vi "ResultsDB Insert Results Data - Copy.vi"(6 "Results NameList":string, 7 "Total_OK/NG":string, 8 "error in (no error)":errorcluster, 9 "Results List":string, 10 "StationName":string, 11 "MainBarcode":string) -> (0 "error out":errorcluster, 3 "CMD":string)   [LabVIEW 2021, in "SQLite.lvclass"]
doc: "写入每一步的测试结果到Results表格。\n写入原理：先检测已经保存了几个结果数据，然后依次附加到结果数据列上。\n# 2020-6-8 14:05:45"
uses:
  SQLite.lvclass
  Y:/UTP_2023/Source_Public/DataBase/Top DB/Top DB.lvclass
  <vilib>/Utility/error.llb/Trim Whitespace.vi
  SQLite.lvclass/SQLite.ctl
  <userlib>/LabSQL/LabSQL.lvlib
  vi.lib_New/TopPath/TopPath.lvlib
  <userlib>/sushu/sushu.lvlib
panel:
  out "Update CMD 3":string
  out "Update CMD 2":string
  out "Update CMD":string
  out "EmptyResultColumnIndex":i32
  out "FirstRow":string[](array[string])
  out "source":string
  out "match substring":string
  out "number (0 to 1)":dbl
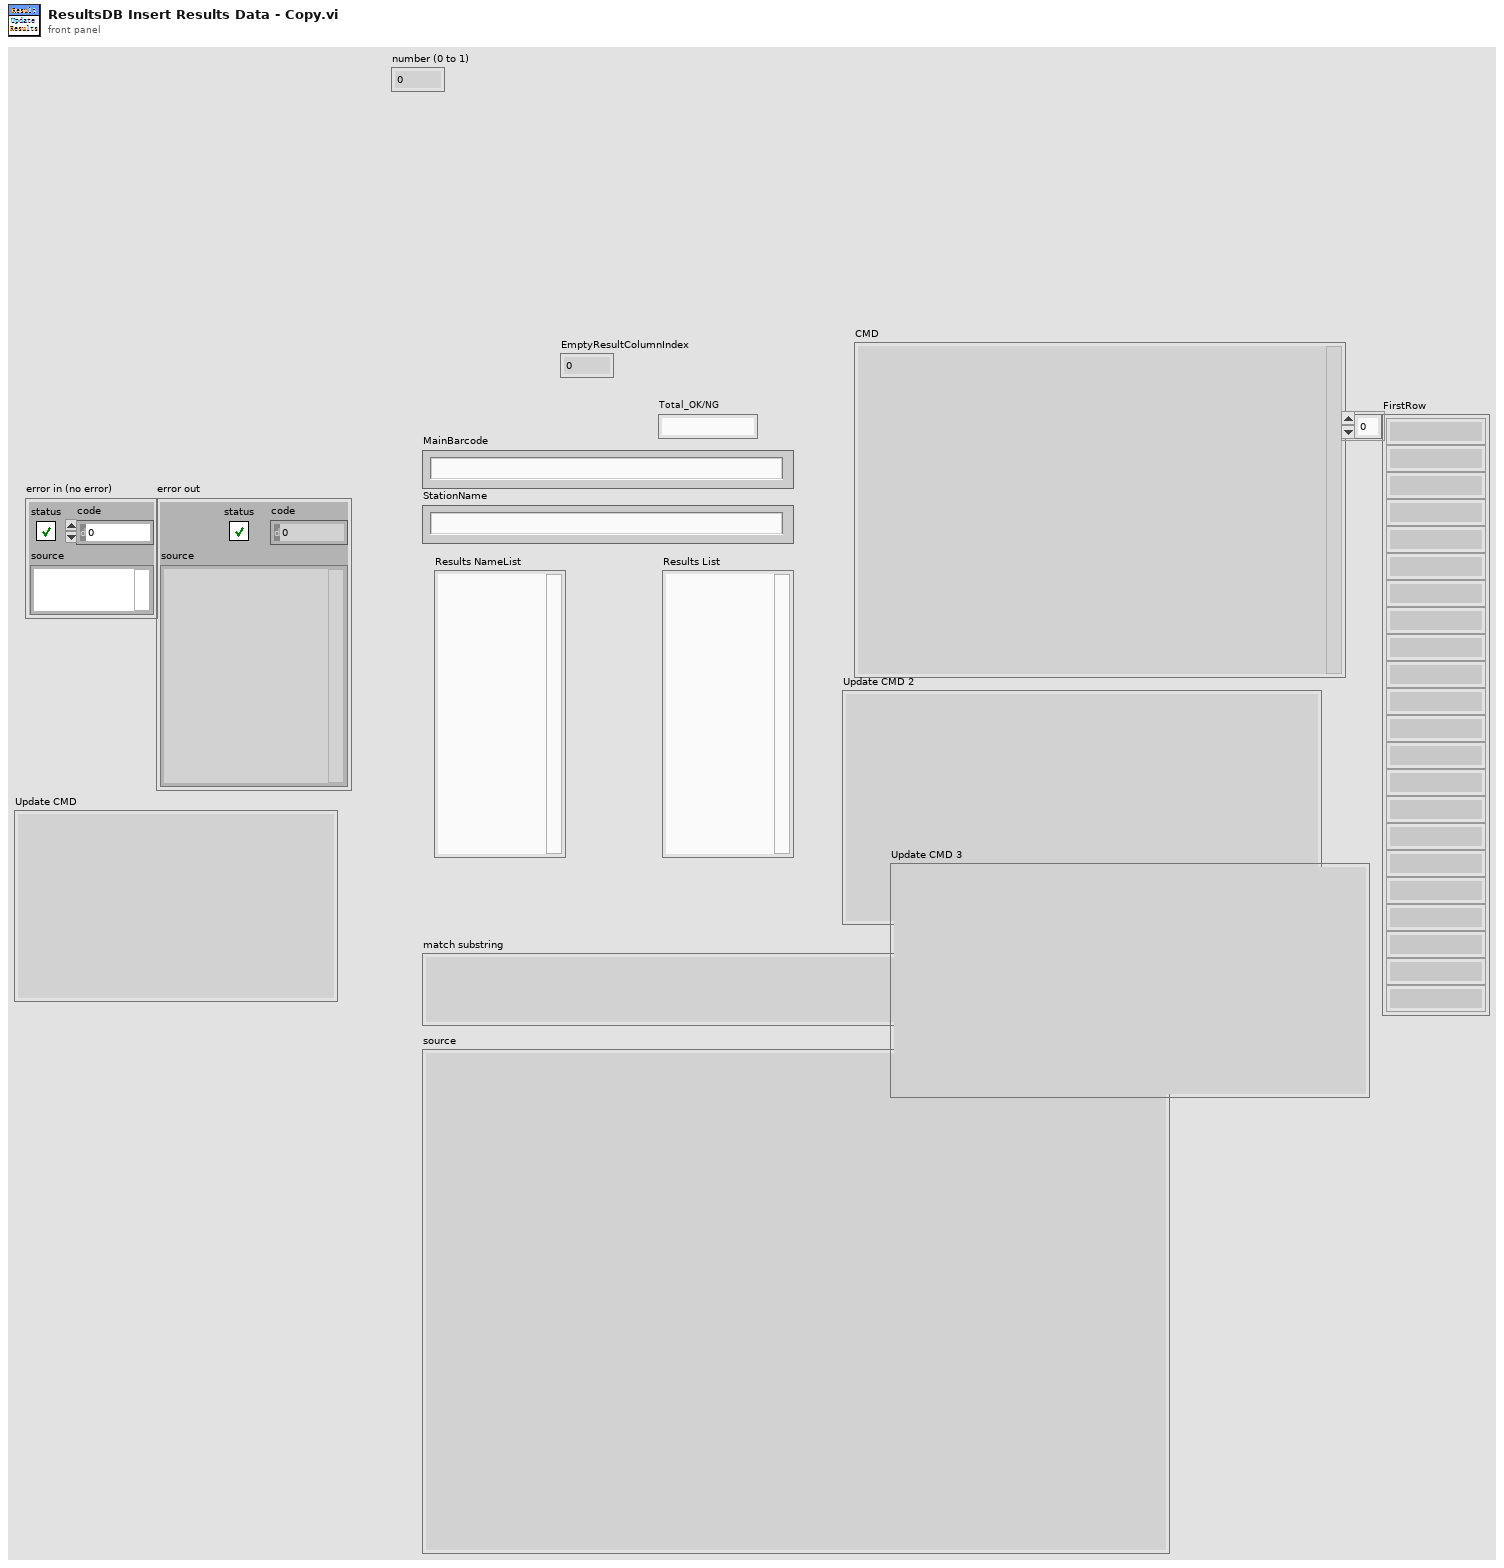
[diagram p1: front panel]
types:
  T1 = cluster{"Core":cluster{"Current VI Reference":refnum<vi>, "Close Panel on Exit?":bool}, "VI Name":string, "Row Numbers":string, "Update?":bool, "CMD":string, "ResultStartindex":i32, "EmptyResultColumnIndex":i32}
  T2 = enum16{"Other", "SQL2008", "SQLite", "Access", "MySQL"}
  T3 = typedef "TopPath.lvlib/Top Path.ctl" = cluster{"LV Source":path, "FilePath":path, "Data":path}
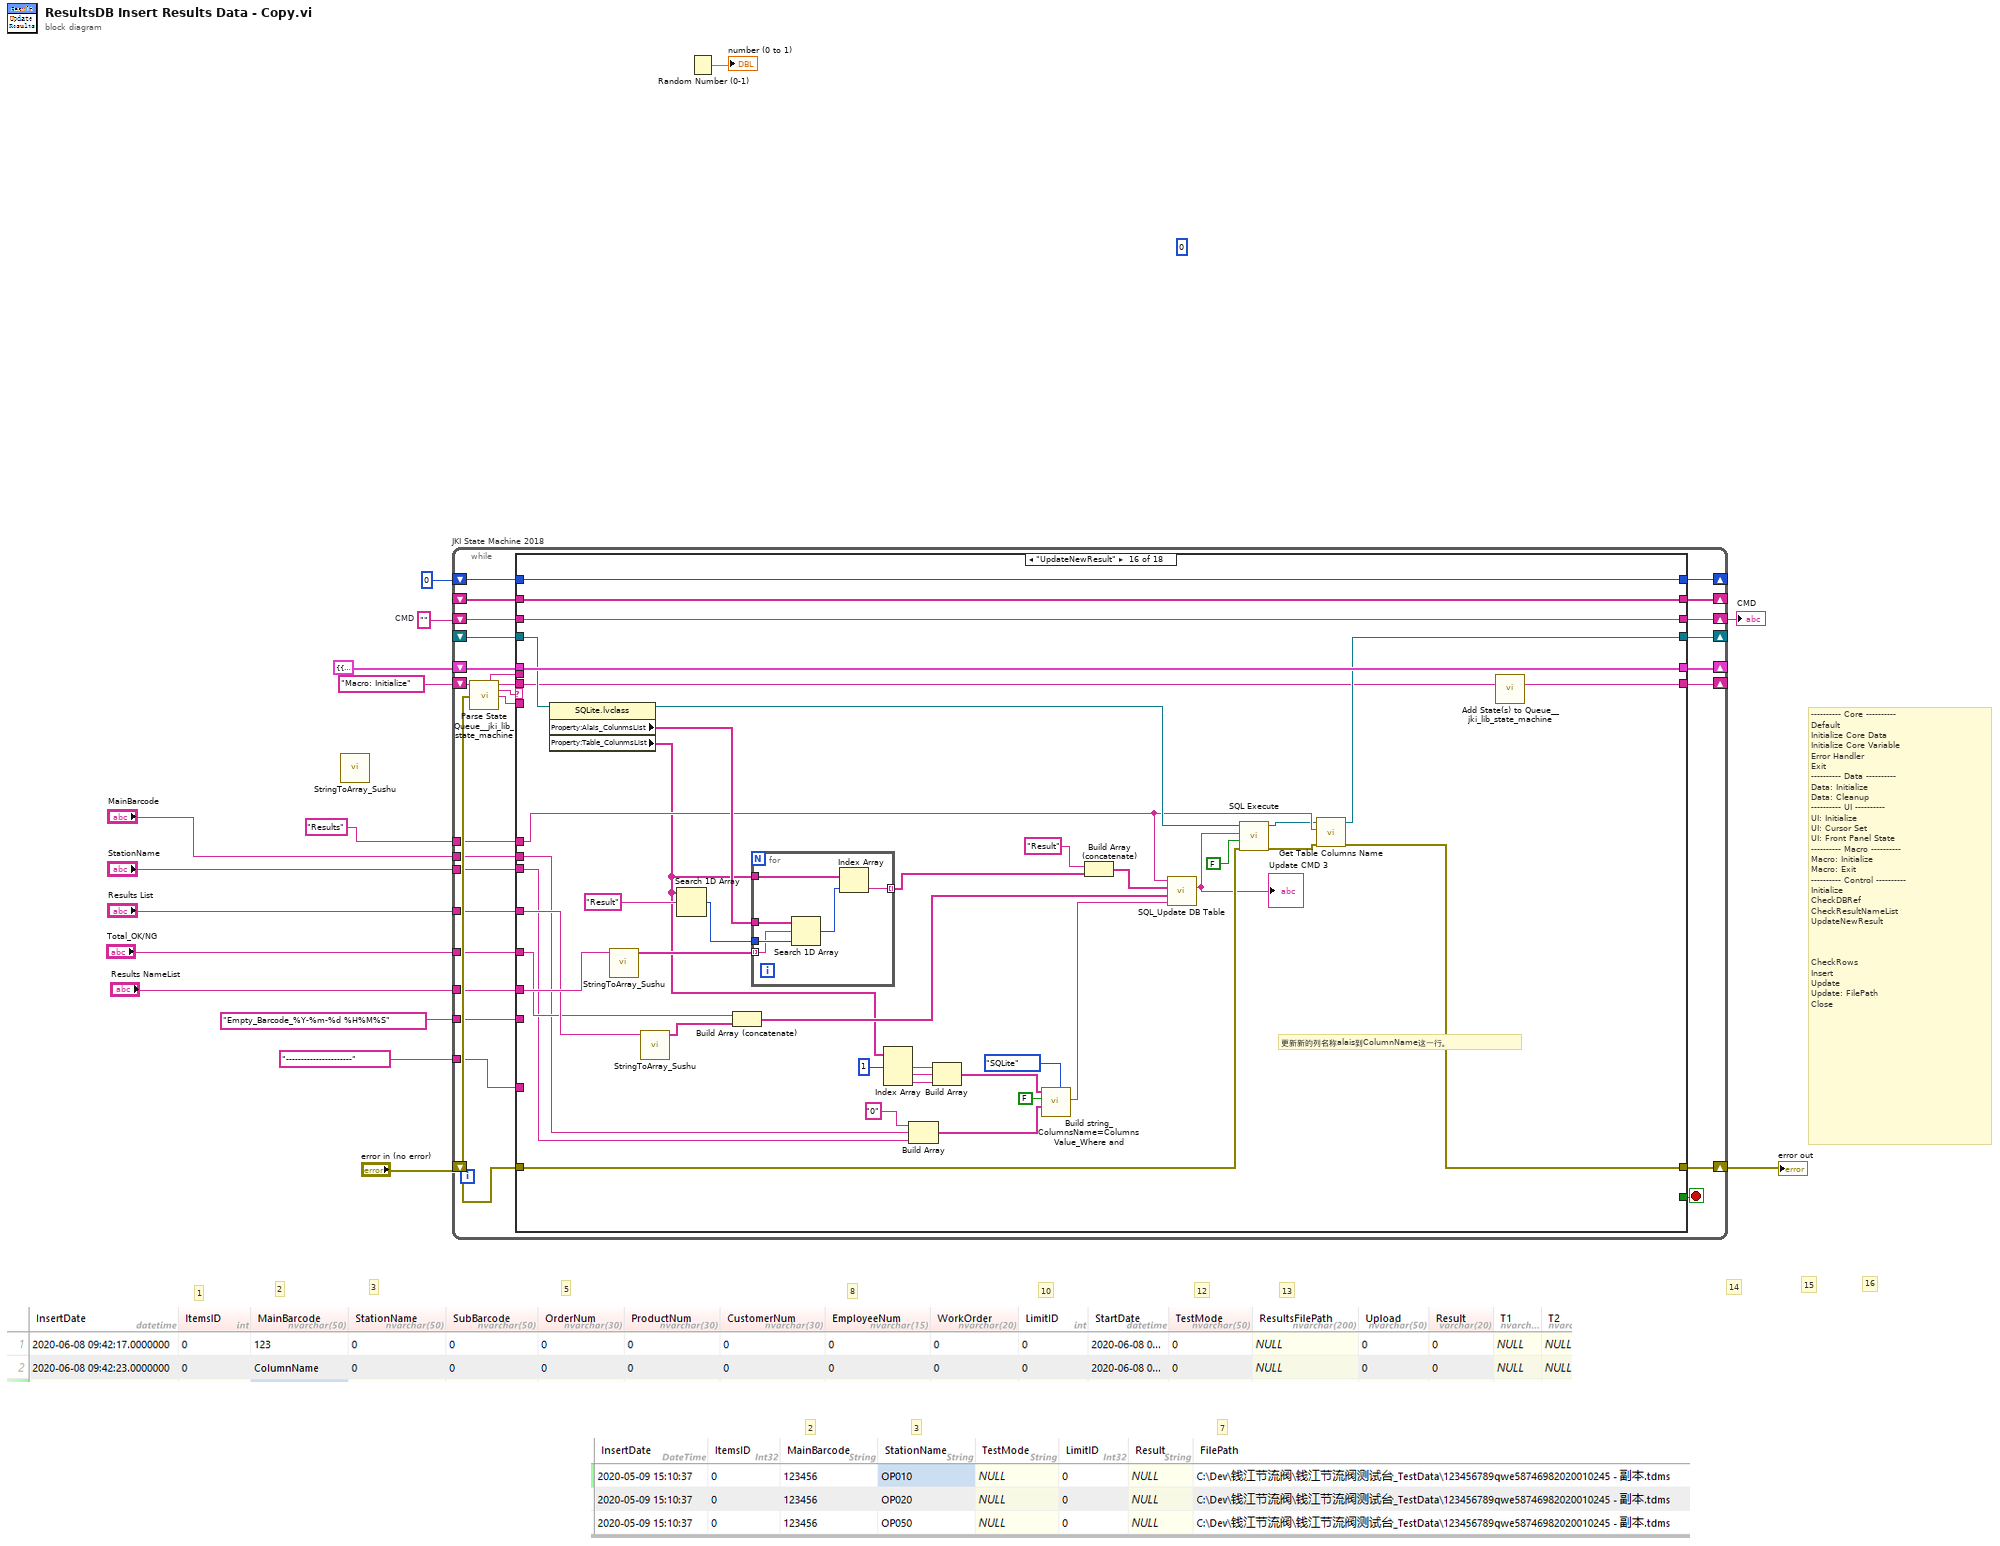
[diagram p0: block diagram]
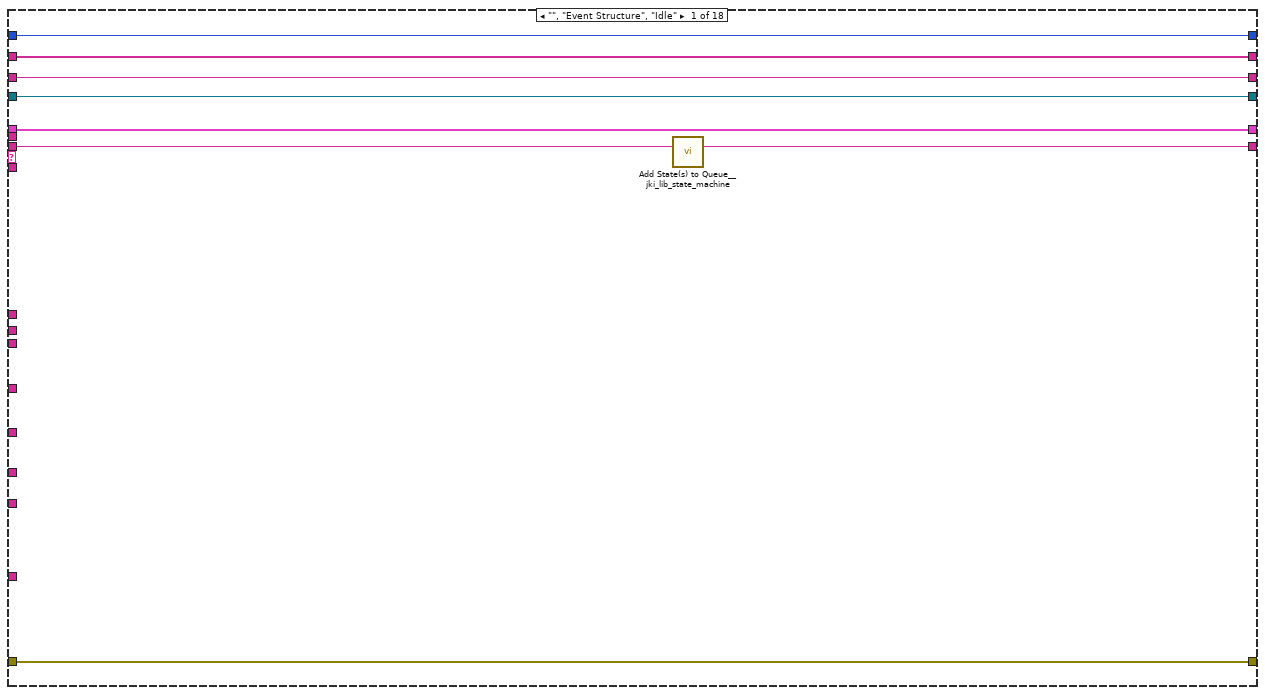
[diagram p2: hidden frame]
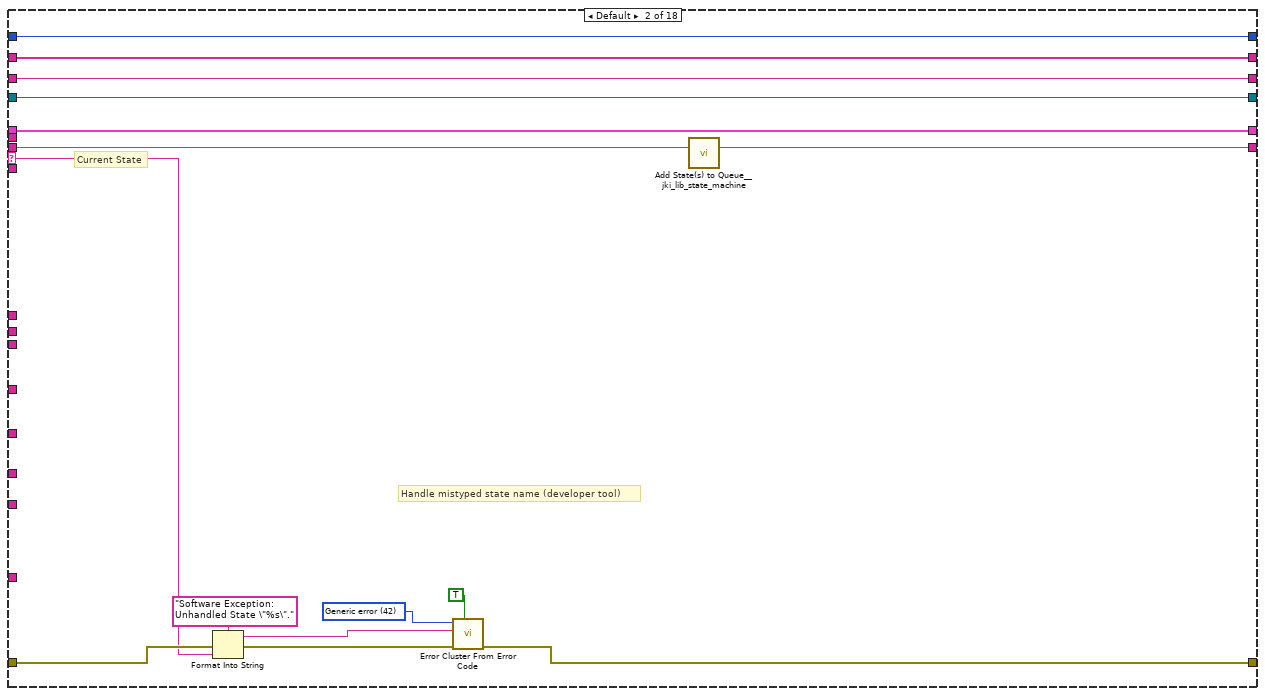
[diagram p3: hidden frame]
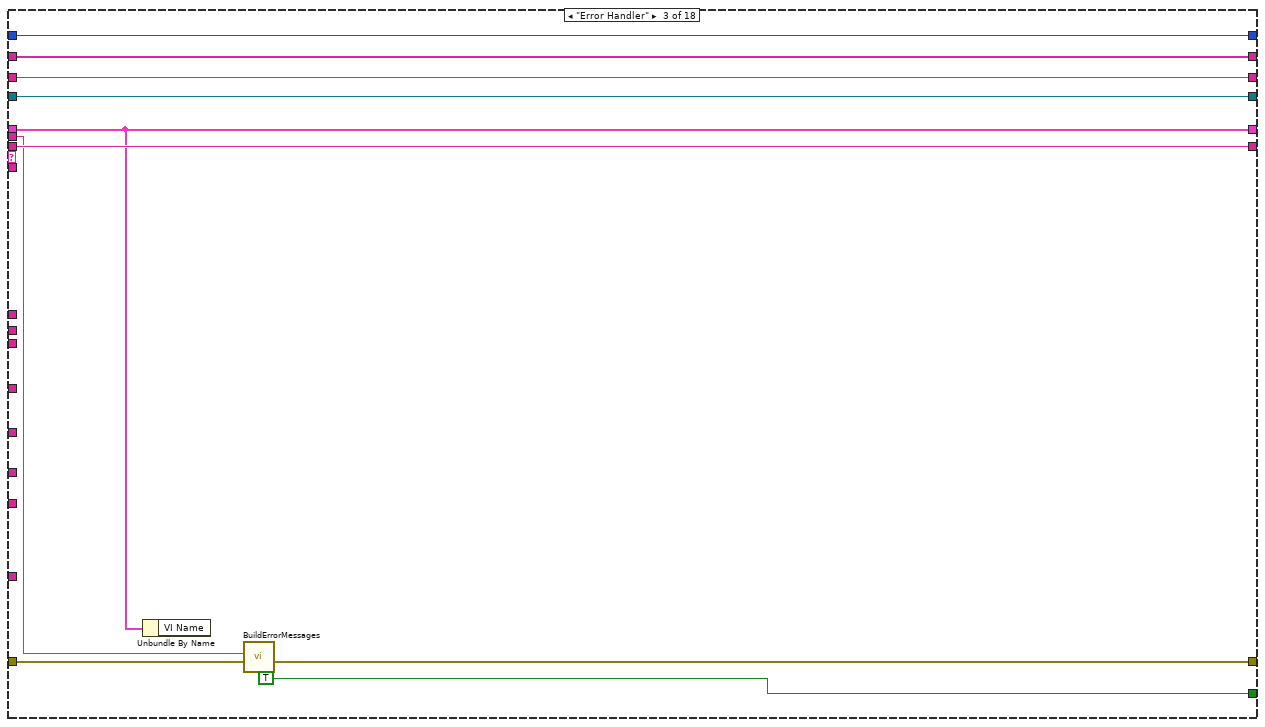
[diagram p4: hidden frame]
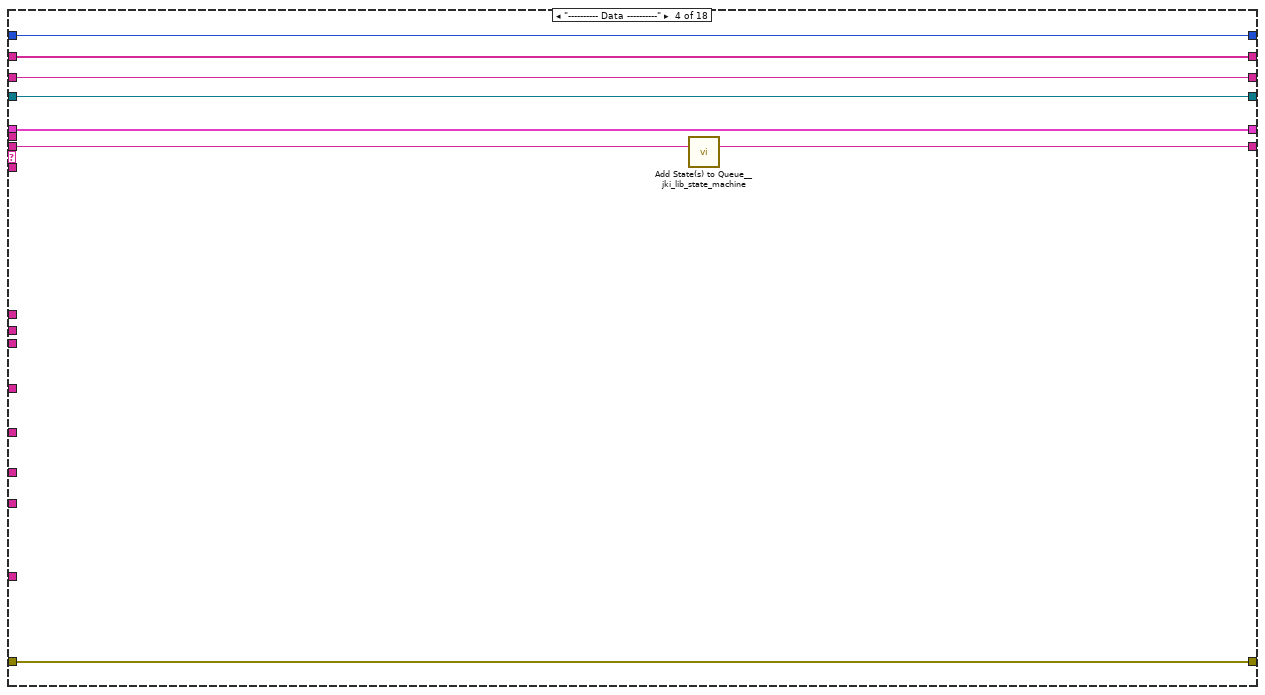
[diagram p5: hidden frame]
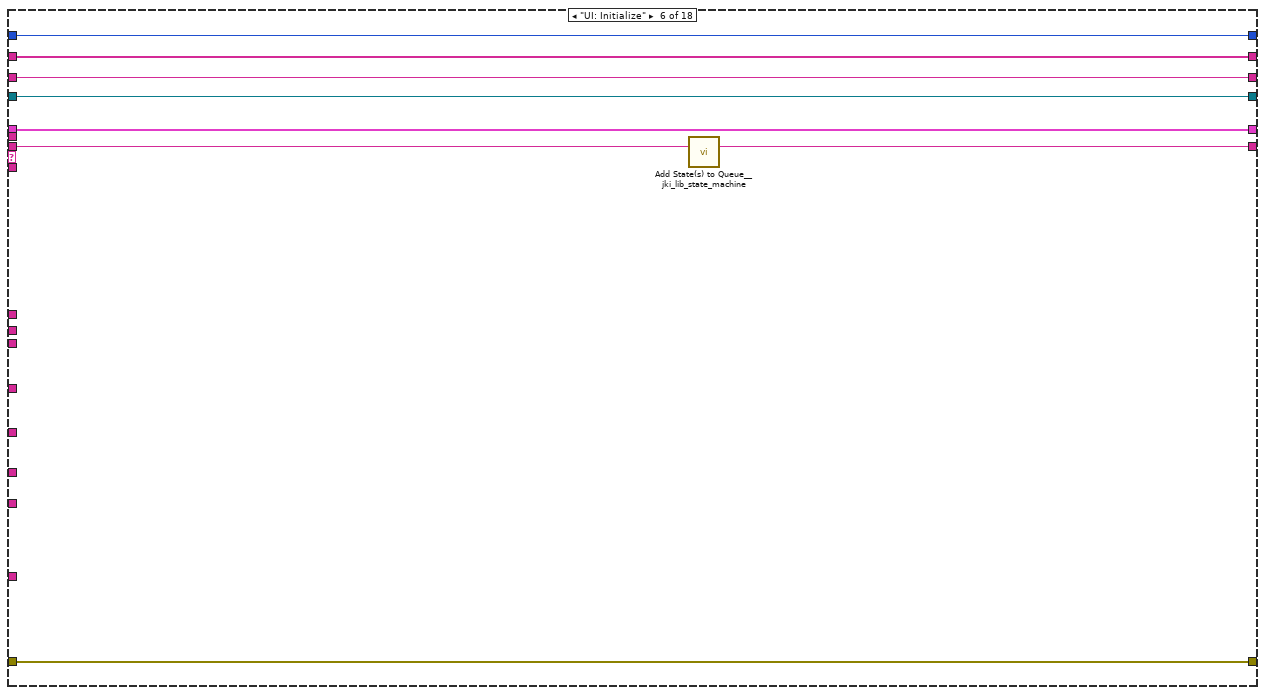
[diagram p7: hidden frame]
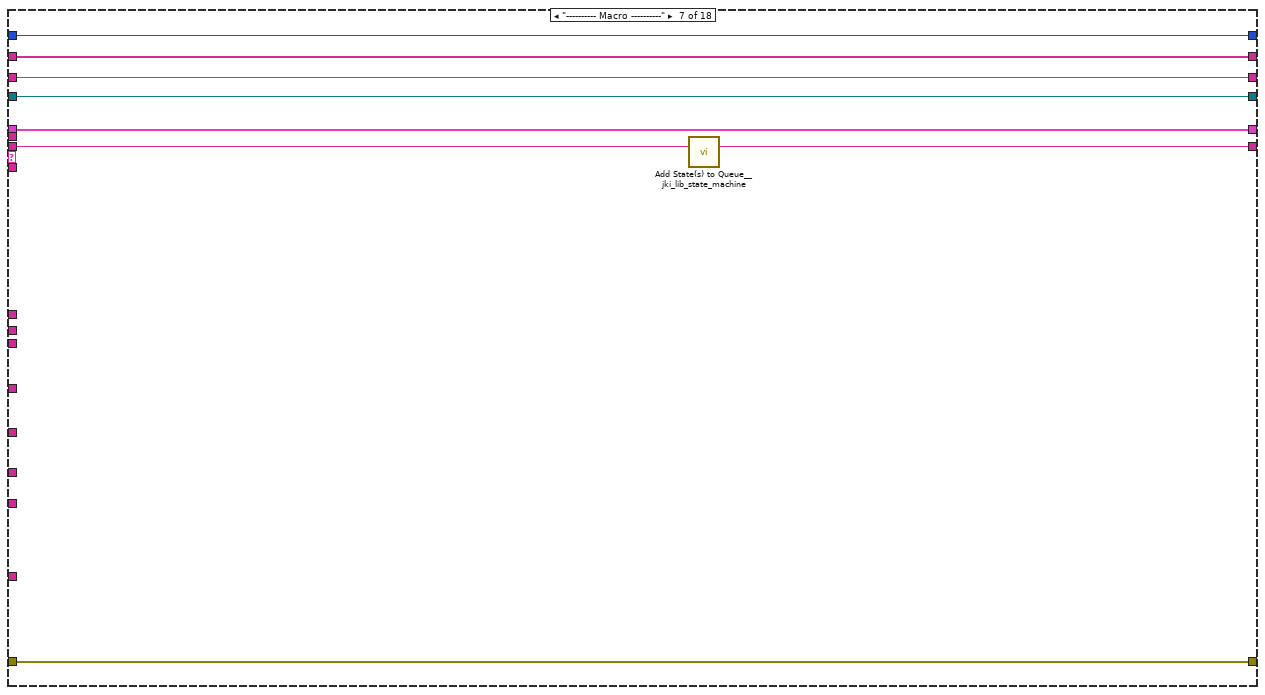
[diagram p8: hidden frame]
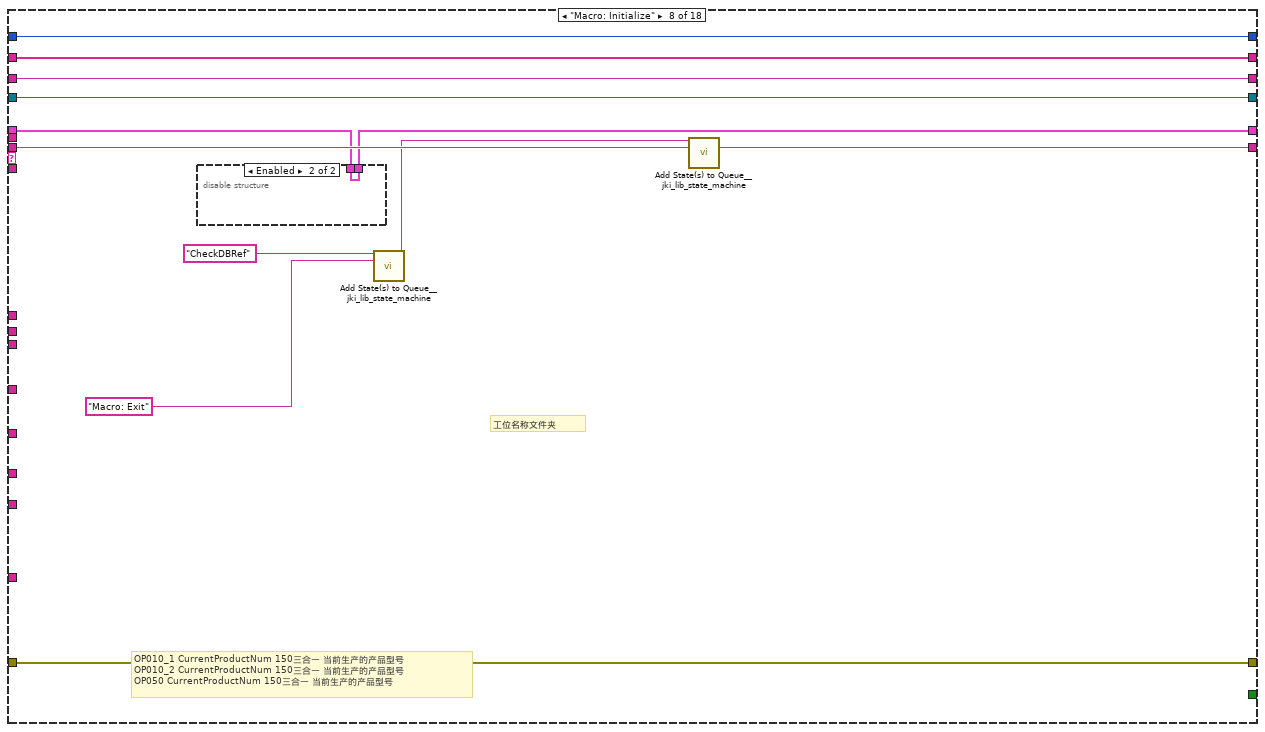
[diagram p9: hidden frame]
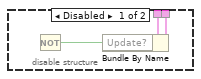
[diagram p10: hidden frame]
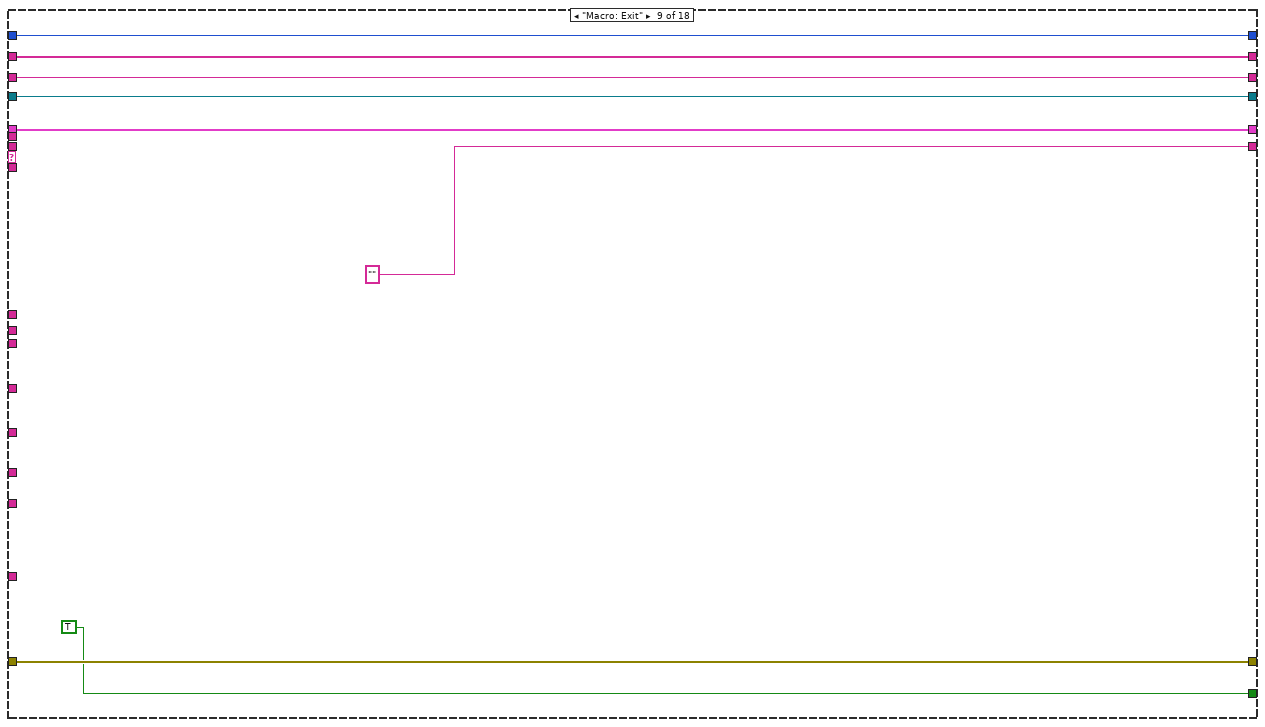
[diagram p11: hidden frame]
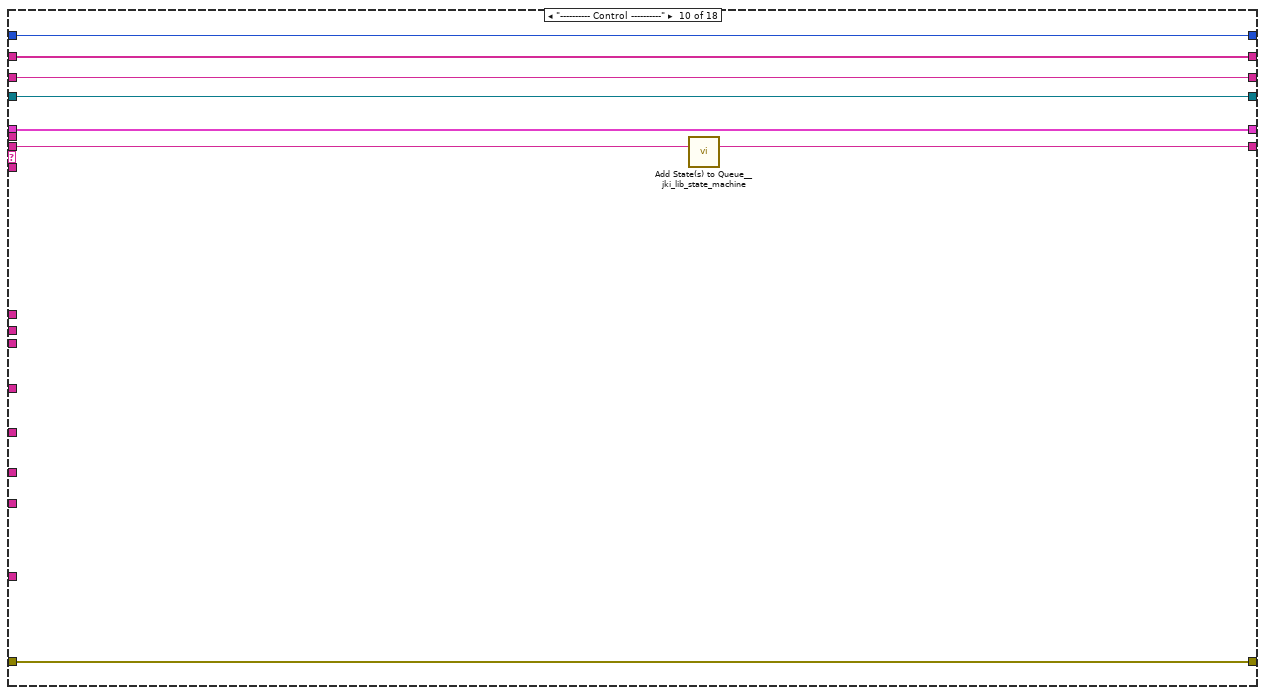
[diagram p12: hidden frame]
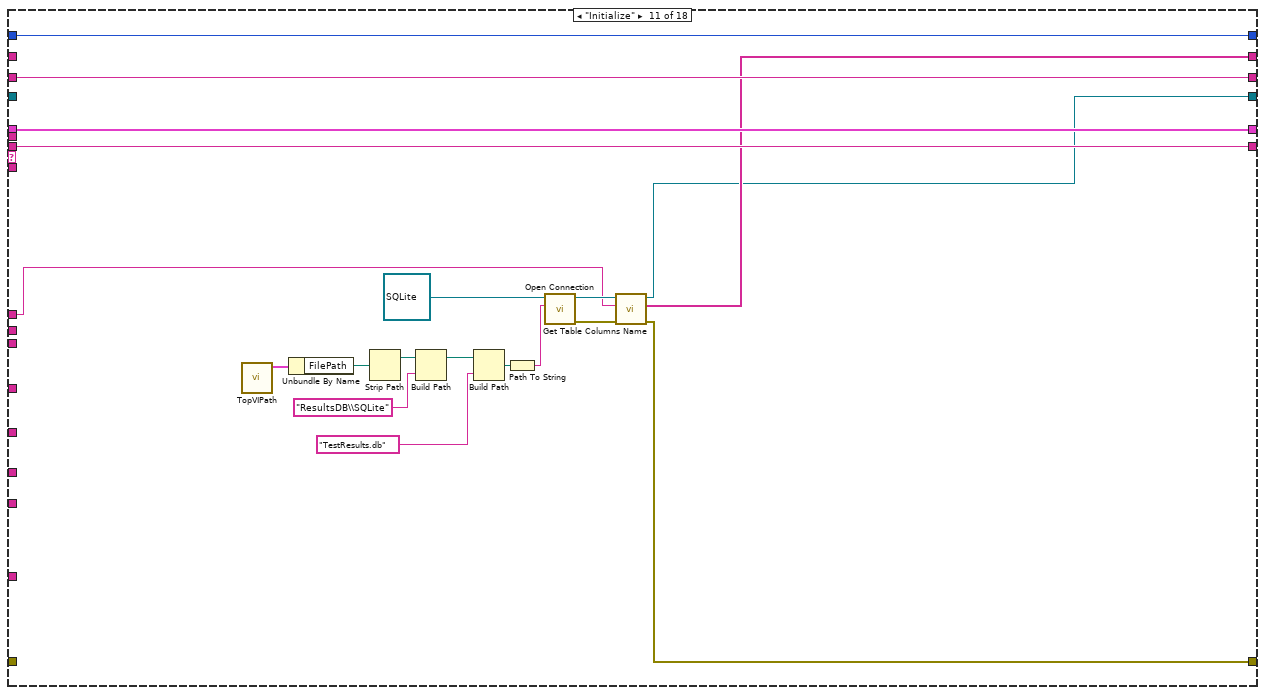
[diagram p13: hidden frame]
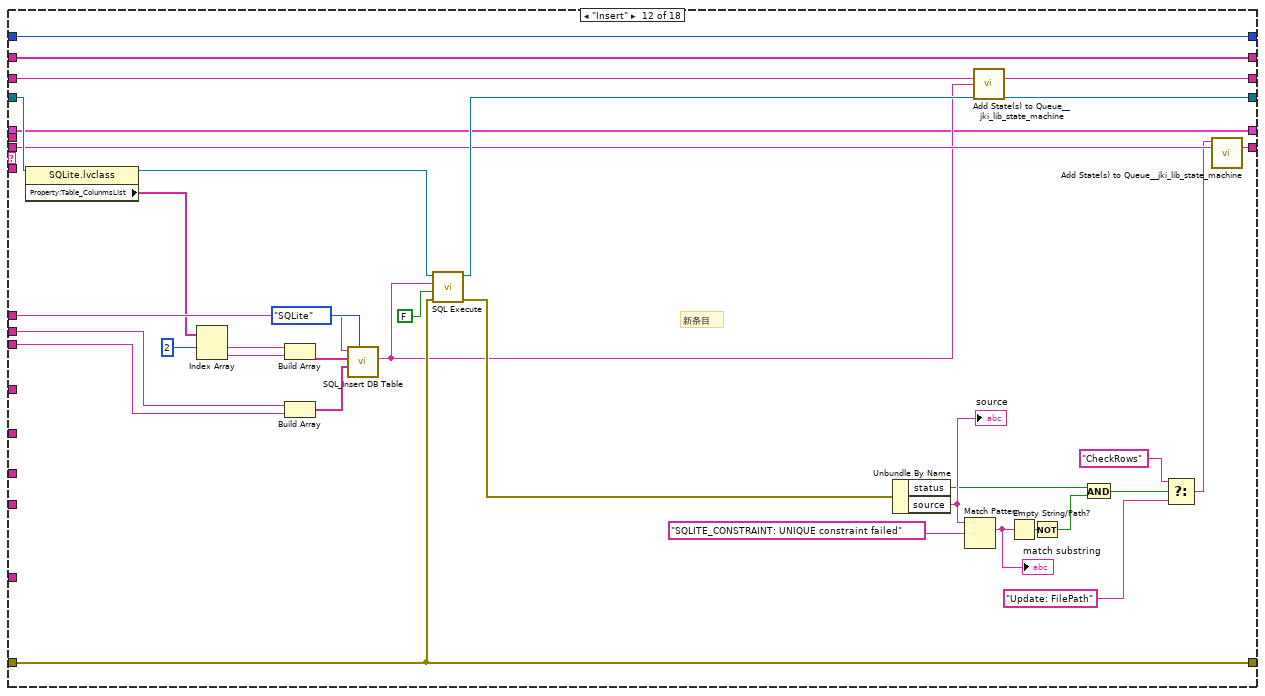
[diagram p14: hidden frame]
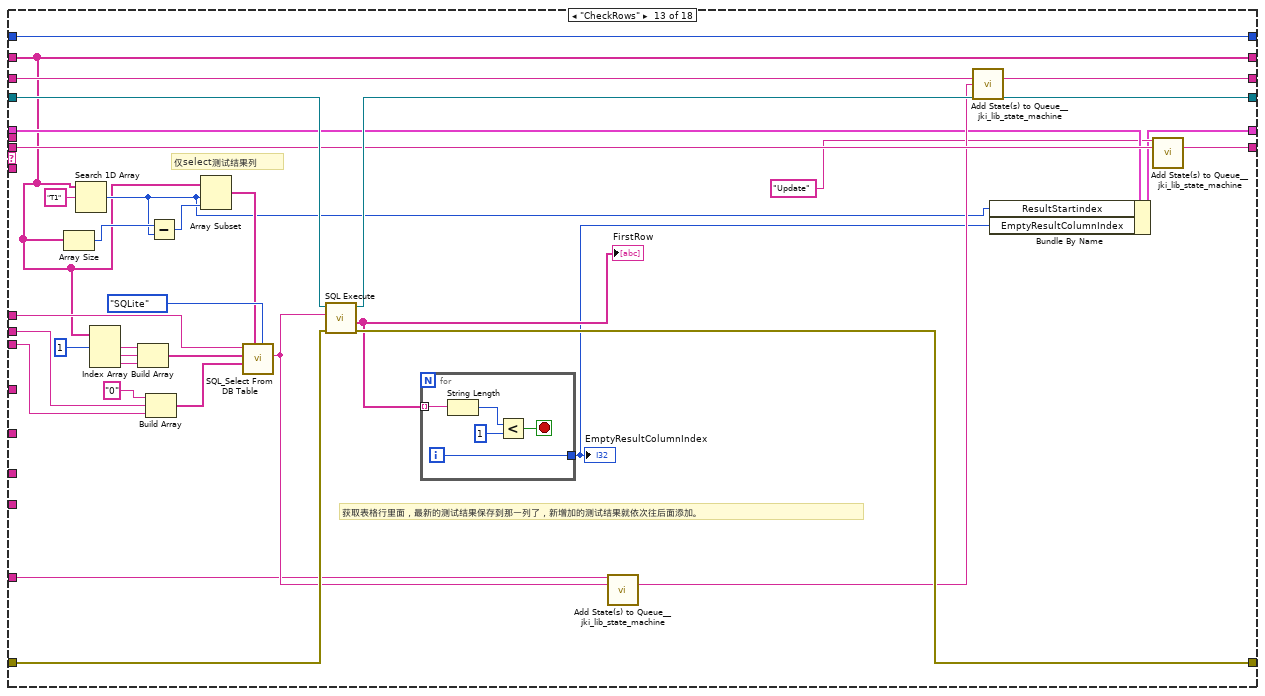
[diagram p15: hidden frame]
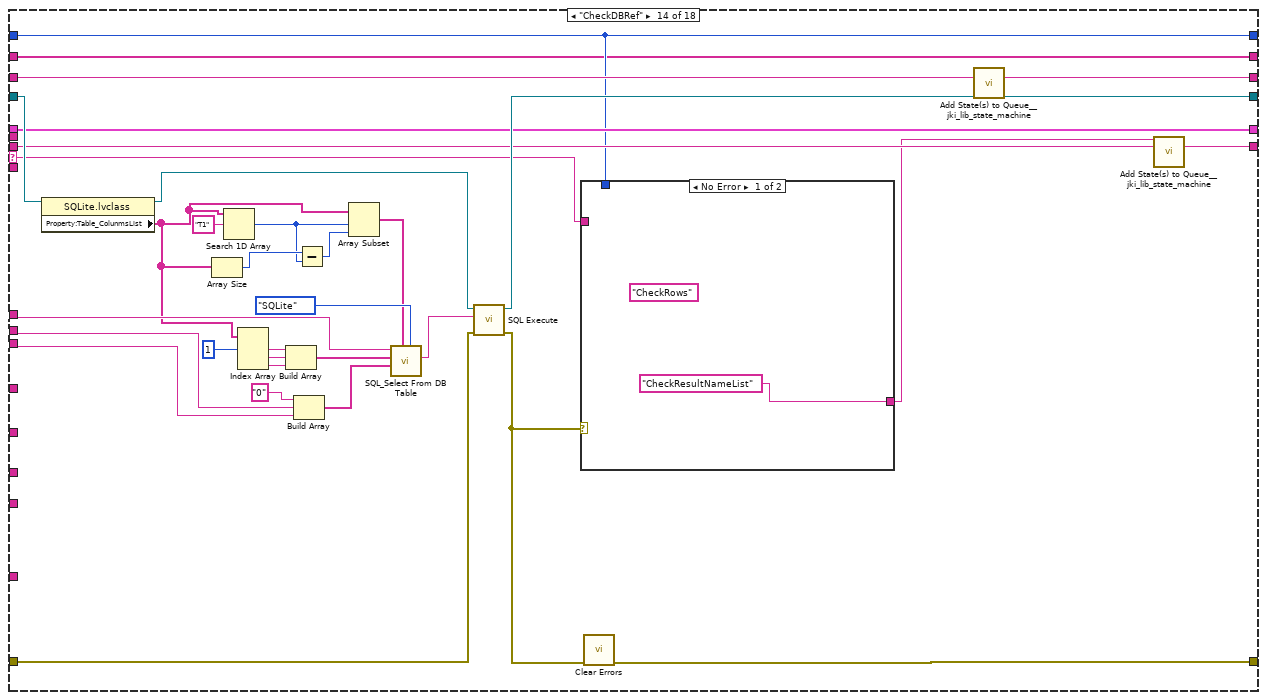
[diagram p16: hidden frame]
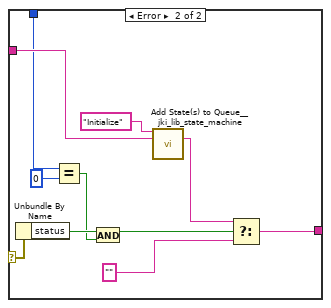
[diagram p17: hidden frame]
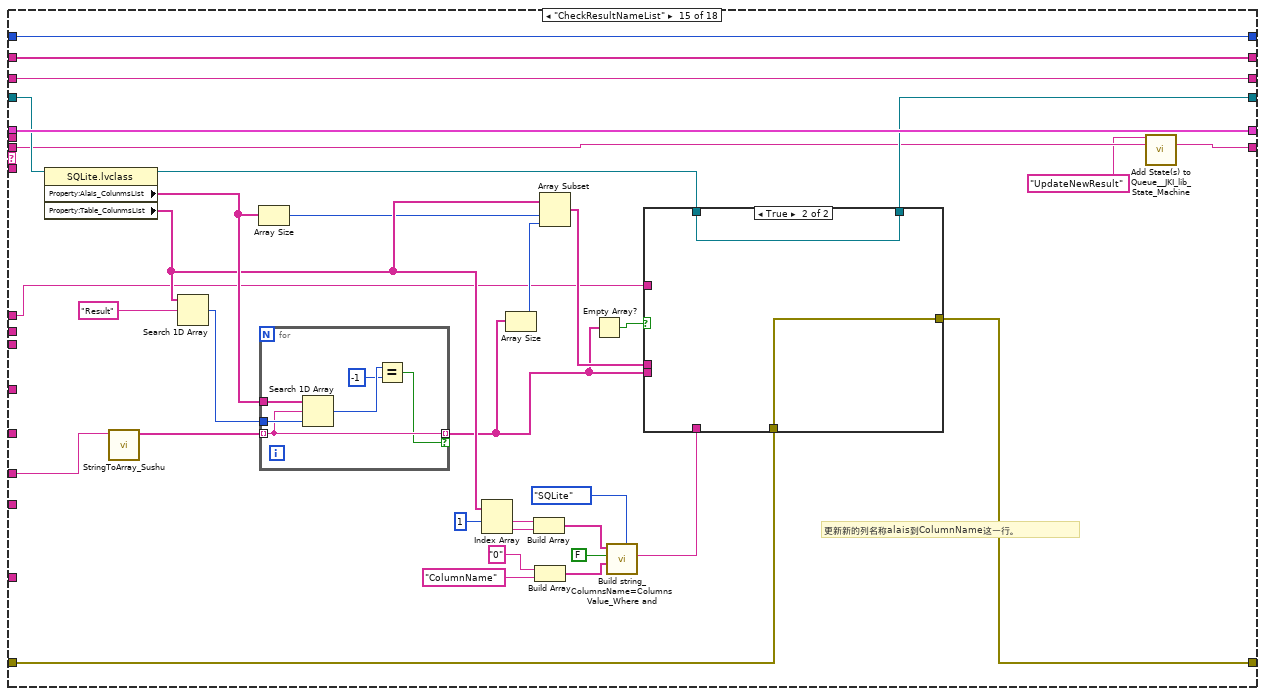
[diagram p18: hidden frame]
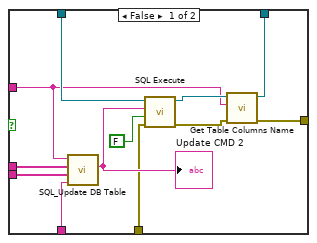
[diagram p19: hidden frame]
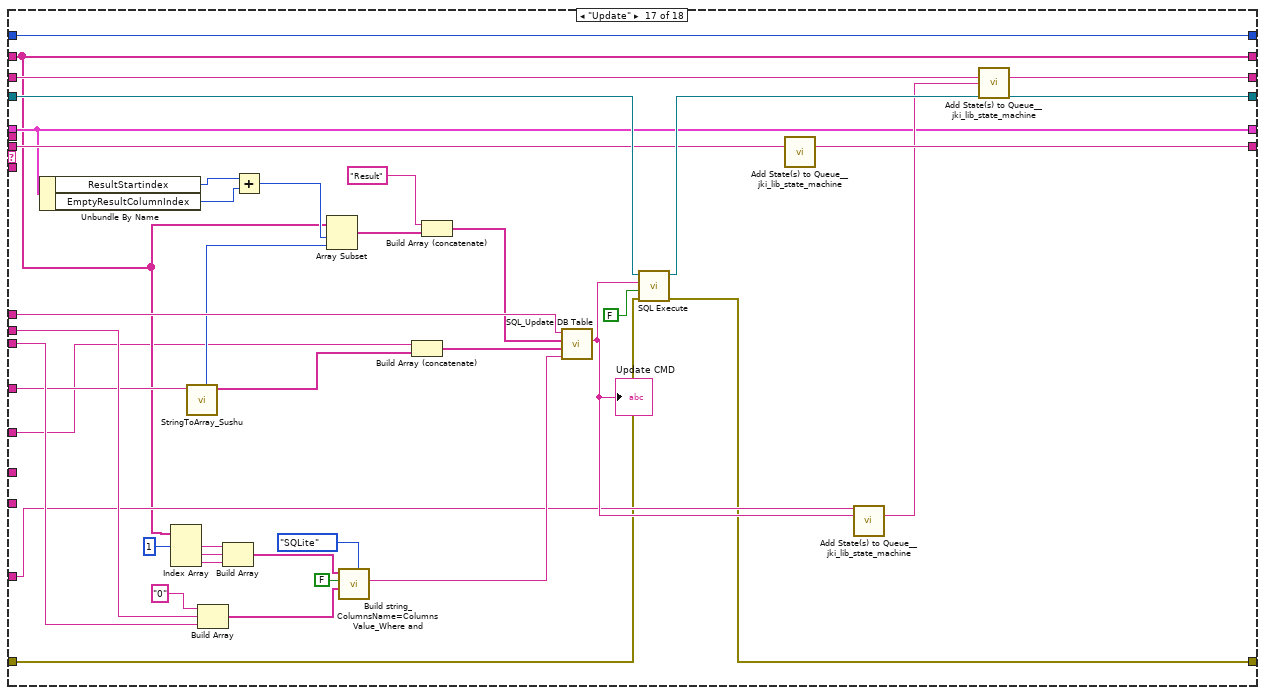
[diagram p20: hidden frame]
diagram:
  w9 = ""  # CMD
  (unwired) 0 ("index (row)")
  # "16"
  # "15"
  # "14"
  # "13"
  # "12"
  # "10"
  # "8"
  # "5"
  # "3"
  # "2"
  # "1"
  # "---------- Core ----------\nDefault\nInitialize Core Data\nInitialize Core Variable\nError Handler\nExit\n---------- Data ----------\nData: Initialize\nData: Cleanup\n---------- UI ----------\nUI: Initialize\nUI: Cursor Set\nUI: Front Panel State\n---------- Macro ----------\nMacro: Initialize\nMacro: Exit\n---------- Control ----------\nInitialize\nCheckDBRef\nCheckResultNameList\nUpdateNewResult\n\n\n\nCheckRows\nInsert\nUpdate\nUpdate: FilePath\nClose"
  # "7"
  # "3"
  # "2"
  n1 = call <userlib>:"StringToArray_Sushu.vi"() -> ()  [unwired: 8 in, 4 out]
  n2 = while "JKI State Machine 2018" {
    shift-right: [w37] -> _
    shift-left: T1 {"Core"={"Current VI Reference"=refnum, "Close Panel on Exit?"=FALSE}, "VI Name"="", "Row Numbers"="", "Update?"=FALSE, "CMD"="", "ResultStartindex"=0, "EmptyResultColumnIndex"=0} ("Data") -> [w36]
    shift-right: [w40] -> w3
    shift-left: "error in (no error)" -> [w35]
    shift-right: [w39] -> _
    shift-left: "Macro: Initialize" -> [w41]
    shift-right: [w33] -> _
    shift-left: _ -> [w34]
    tunnel: "StationName" -> [w31]
    tunnel: "MainBarcode" -> [w30]
    tunnel: "Results" ("TableName") -> [w29]
    tunnel: "Empty_Barcode_%Y-%m-%d %H%M%S" ("time format string (%c)") -> [w28]
    shift-right: [w27] -> w7
    shift-left: w9 -> [w26]
    tunnel: "----------------------" ("State(s) in (\"\")") -> [w25]
    tunnel: "Results List" -> [w24]
    shift-right: [w22] -> _
    shift-left: _ -> [w23]
    shift-right: [w21] -> _
    shift-left: 0 ("y") -> [w20]
    tunnel: "Total_OK/NG" -> [w19]
    tunnel: "Results NameList" -> [w17]
    stop <- w38 stop-if-true
    n3 = call <vilib>:"Parse State Queue__jki_lib_state_machine.vi"("State Queue"=w41, "Error In (no error)"=w35) -> ("Previous State"=w18:string, "Remaining States"=w43:string, "Current State"=w32:string, "Arguments"=w42:string)  [unwired: 10 in]
    n4 = case shown="\"UpdateNewResult\"" w32 {
      selector: w32 -> [_ w56 _ _ _ _ _ _ _ _ _ _ _ w239 _ _ _ _]
      tunnel: w43 -> [w51 w60 w75 w84 w88 w99 w107 w119 _ w139 w158 w170 w214 w252 w278 w355 w409 w425]
      tunnel: w42 -> [_ _ _ _ _ _ _ _ _ _ _ _ _ _ _ _ _ _]
      tunnel: w36 -> [w48 w58 w73 w81 w89 w97 w104 w115 w130 w136 w157 w163 w200 w241 w310 w371 w392 w424]
      tunnel: [w49 w62 w70 w82 w91 w96 w105 w116 w131 w137 w143 w180 w212 w235 w283 w358 w384 w419] -> w40
      tunnel: w35 -> [w49 w61 w71 w82 w91 w96 w105 w116 w131 w137 _ w180 w213 w251 w301 w362 w385 w420]
      tunnel: [w50 w59 w75 w83 w88 w98 w106 w118 "" w138 w158 w171 w215 w253 w279 w356 w410 w425] -> w39
      tunnel: [_ _ TRUE _ _ _ _ _ TRUE _ _ _ _ _ _ _ _ _] -> w38
      tunnel: [w48 w58 w73 w81 w89 w97 w104 w111 w130 w136 w157 w163 w197 w241 w310 w371 w392 w424] -> w37
      tunnel: w34 -> [w47 w55 w74 w80 w90 w95 w103 w117 w129 w135 _ w183 w217 w255 w309 w370 w413 w418]
      tunnel: [w47 w55 w74 w80 w90 w95 w103 w117 w129 w135 w140 w182 w216 w254 w284 w359 w412 w417] -> w33
      tunnel: w18 -> [_ _ w72 _ _ _ _ _ _ _ _ _ _ _ _ _ _ _]
      tunnel: w31 -> [_ _ _ _ _ _ _ _ _ _ _ w184 w218 w256 _ w331 w414 _]
      tunnel: w30 -> [_ _ _ _ _ _ _ _ _ _ _ w185 w219 w257 _ w332 w415 _]
      tunnel: w29 -> [_ _ _ _ _ _ _ _ _ _ w144 w186 w220 w258 w282 w357 w416 _]
      tunnel: w28 -> [_ _ _ _ _ _ _ _ _ _ _ _ _ _ _ _ _ _]
      tunnel: w26 -> [w46 w54 w69 w79 w87 w94 w102 w112 w126 w134 w156 w166 w210 w249 w308 w369 w397 w423]
      tunnel: [w46 w54 w69 w79 w87 w94 w102 w112 w126 w134 w156 w165 w211 w250 w308 w369 w398 w423] -> w27
      tunnel: w25 -> [_ _ _ _ _ _ _ _ _ _ _ _ w207 _ _ _ w394 _]
      tunnel: w24 -> [_ _ _ _ _ _ _ _ _ _ _ _ _ _ _ w350 w393 _]
      tunnel: w23 -> [w45 w53 w68 w78 w86 w93 w101 w109 w125 w133 _ w160 w194 w233 w307 w368 w383 w422]
      tunnel: [w45 w53 w68 w78 w86 w93 w101 w109 w125 w133 w141 w160 w194 w233 w307 w368 w383 w422] -> w22
      tunnel: w20 -> [w44 w52 w67 w77 w85 w92 w100 w108 w124 w132 w142 w162 w193 w238 w306 w367 w382 w421]
      tunnel: [w44 w52 w67 w77 w85 w92 w100 w108 w124 w132 w142 w162 w193 w238 w306 w367 w382 w421] -> w21
      tunnel: w19 -> [_ _ _ _ _ _ _ _ _ _ _ _ _ _ _ w348 w380 _]
      tunnel: w17 -> [_ _ _ _ _ _ _ _ _ _ _ _ _ _ w285 w360 _ _]
      frame "", "Event Structure", "Idle" {
        n5 = call <vilib>:"Add State(s) to Queue__jki_lib_state_machine.vi"("State(s) in (\"\")"=w51) -> ("States Out"=w50:string)  [unwired: 14 in]
      }
      frame Default {
        w65 = 42 items=["No error", "Argument error", "Memory is full", "Out of zone", "End of file", "File already open", "Generic file I/O error", "File not found", "File permission error", "Disk is full", "Duplicate path", "Too many files open", "System feature not enabled", "Resource file not found", "Cannot add resource", "Resource not found", "Image not found", "Image memory error", "Pen does not exist", "Config type invalid", "Config token not found", "Config parse error", "Config memory error", "Bad external code format", "Bad external code offset", "External code not present", "Null window", "Destroy window error", "Null menu", "Print aborted", "Bad print record", "Print driver error", "Windows error during printing", "Memory error during printing", "Print dialog error", "Generic print error", "Invalid device refnum", "Device not found", "Device parameter error", "Device unit error", "Cannot open device", "Device call aborted", "Generic error", "Cancelled by user", "Object ID too low", "Object ID too high", "Object not in heap", "Unknown heap", "Unknown object (invalid DefProc)", "Unknown object (DefProc not in table)", "Message out of range", "Invalid (null) method", "Unknown message", "Manager call not supported", "Bad address", "Network operation in progress", "Network operation timed out", "Connection is busy", "Network attribute not supported", "Network error", "Address in use", "System out of memory", "Connection aborted", "Connection refused", "Not connected", "Already connected", "Connection closed", "Initialization error (interapplication manager)", "Bad occurrence", "Wait on unbound occurrence handler", "Occurrence queue overflow", "Datalog type conflict", "Unused", "Unrecognized type (interapplication manager)", "Memory corrupt", "Failed to make temporary DLL", "Old CIN version", "Drag socket not found", "Failed to load drop-object", "Failed to register OLE object", "Failed to release OLE object", "Format specifier type mismatch", "Unknown format specifier", "Too few format specifiers", "Too many format specifiers", "Scan failed", "Newer CIN version", "Error converting to variant", "Runtime menu error", "Password tampered", "Variant attribute not found", "Incompatible variant data type", "Event data is not available", "Event Store is not present", "Occurrence is not found", "Event Queue is not created", "Event info is not available", "Refnum passed is NULL", "Error retrieving Class GUID", "Error retrieving CoClass GUID", "Error retrieving TypeLib GUID.", "Bad built application magic bytes.", "Specific driver is different from the specific driver associated with the Logical Name.", "There is no session opened to the class driver.", "Max Error", "MAX - Error with config objects", "MAX - Error loading configuration", "MAX - Group not supported"]
        # "Current State"
        # "Handle mistyped state name (developer tool)"
        n6 = Format Into String(format string="Software Exception: Unhandled State \"%s\"." ("message"), error in=w61, w56) -> (resulting string=w64:string, error out=w63:errorcluster)  [unwired: 1 in]
        n7 = call <vilib>:"Error Cluster From Error Code.vi"("show call chain? (False)"=TRUE, "error in (no error)"=w63, "error message (\"\")"=w64, "error code (0)"=w65) -> ("error out"=w62:errorcluster)  [unwired: 5 in]
        n8 = call <vilib>:"Add State(s) to Queue__jki_lib_state_machine.vi"("State(s) in (\"\")"=w60) -> ("States Out"=w59:string)  [unwired: 14 in]
      }
      frame "Error Handler" {
        n9 = Unbundle By Name(w73) -> ()  [unwired: 1 out]
        n10 = call <userlib>:"BuildErrorMessages.vi"("error in"=w71, "ErrorCase"=w72) -> ("error out (no error)"=w70:errorcluster)  [unwired: 7 in, 2 out]
      }
      frame "---------- Data ----------" {
        n11 = call <vilib>:"Add State(s) to Queue__jki_lib_state_machine.vi"("State(s) in (\"\")"=w84) -> ("States Out"=w83:string)  [unwired: 14 in]
      }
      frame "Data: Initialize" {
      }
      frame "UI: Initialize" {
        n12 = call <vilib>:"Add State(s) to Queue__jki_lib_state_machine.vi"("State(s) in (\"\")"=w99) -> ("States Out"=w98:string)  [unwired: 14 in]
      }
      frame "---------- Macro ----------" {
        n13 = call <vilib>:"Add State(s) to Queue__jki_lib_state_machine.vi"("State(s) in (\"\")"=w107) -> ("States Out"=w106:string)  [unwired: 14 in]
      }
      frame "Macro: Initialize" {
        # "OP010_1\tCurrentProductNum\t150三合一\t当前生产的产品型号\nOP010_2\tCurrentProductNum\t150三合一\t当前生产的产品型号\nOP050\tCurrentProductNum\t150三合一\t当前生产的产品型号"
        # "工位名称文件夹"
        n14 = disable-structure shown="Enabled" {
          disable-tunnel: w115 -> [w122 w123]
          disable-tunnel: [w121 w123] -> w111
          frame Disabled {
            n15 = Not() -> (.not. x?=w120:bool)  [unwired: 1 in]
            n16 = Bundle By Name(cluster=w122, "Update?"=w120) -> (w121:T1)
          }
          frame Enabled {
          }
        }
        n17 = call <vilib>:"Add State(s) to Queue__jki_lib_state_machine.vi"("State(s) in Front (\"\")"="CheckDBRef" ("State(s) in Front (\"\")"), "State(s) in (\"\")"="Macro: Exit") -> ("States Out"=w114:string)  [unwired: 13 in]
        n18 = call <vilib>:"Add State(s) to Queue__jki_lib_state_machine.vi"("State(s) in Front (\"\")"=w114, "State(s) in (\"\")"=w119) -> ("States Out"=w118:string)  [unwired: 13 in]
      }
      frame "Macro: Exit" {
      }
      frame "---------- Control ----------" {
        n19 = call <vilib>:"Add State(s) to Queue__jki_lib_state_machine.vi"("State(s) in (\"\")"=w139) -> ("States Out"=w138:string)  [unwired: 14 in]
      }
      frame "Initialize" {
        n20 = call "TopVIPath.vi"() -> ("TopPath"=w145:T3)  [unwired: 10 in, 1 out]
        n21 = Unbundle By Name(w145) -> ("FilePath"=w155:path)
        n22 = Strip Path(path=w155) -> (stripped path=w154:path)  [unwired: 1 out]
        n23 = Build Path(base path=w154, name or relative path="ResultsDB\\SQLite") -> (appended path=w152:path)
        n24 = Build Path(base path=w152, name or relative path="TestResults.db") -> (appended path=w150:path)
        n25 = Path To String(path=w150) -> (string=w149:string)
        n26 = call-dynamic "Open Connection.vi"("ConnectionString"=w149, "HostDB in"=refnum<class "SQLite.lvclass"> refnum ("SQLite.lvclass")) -> ("error out"=w147:errorcluster, "HostDB out"=w148:refnum<class "SQLite.lvclass">)  [unwired: 8 in]
        n27 = call-dynamic "Get Table Columns Name.vi"("error in (no error)"=w147, "TableName"=w144, "HostDB in"=w148) -> ("error out"=w143:errorcluster, "Table_ColunmsList"=w141:string[], "HostDB out"=w140:refnum<class "SQLite.lvclass">)  [unwired: 4 in, 2 out]
      }
      frame "Insert" {
        # "新条目"
        n28 = property class="SQLite.lvclass"(reference=w183) -> (reference out=w161:refnum<class "SQLite.lvclass">, "Property:Table_ColunmsList"=w159:string[])  [unwired: 1 in, 1 out]
        n29 = Index Array(array=w159, index #1=2 ("index")) -> (element #1=w191:string, element #2=w192:string)  [unwired: 1 in]
        n30 = Build Array(w191, w192) -> (w189:string[])
        n31 = Build Array(w185, w184) -> (w188:string[])
        n32 = call <userlib>:"SQL_Insert DB Table.vi"("DB Type"=T2."SQLite", "ColumnsValue"=w188, "ColumnsName"=w189, "Table Name"=w186) -> ("Insert DB String"=w164:string)  [unwired: 7 in]
        n33 = call-dynamic "SQL Execute.vi"("error in (no error)"=w180, "Return Data (T)"=FALSE, "Command Text"=w164, "HostDB in"=w161) -> ("error out"=w167:errorcluster, "HostDB out"=w182:refnum<class "SQLite.lvclass">)  [unwired: 3 in, 3 out]
        n34 = Unbundle By Name(w167) -> ("status"=w176:bool, "source"=w179:string)
        "source" <- w179
        n35 = Match Pattern(string=w179, regular expression="SQLITE_CONSTRAINT: UNIQUE constraint failed") -> (match substring=w177:string)  [unwired: 1 in, 3 out]
        "match substring" <- w177
        n36 = call <vilib>:"Add State(s) to Queue__jki_lib_state_machine.vi"("State(s) in (\"\")"=w166, "State(s) at Back (\"\")"=w164) -> ("States Out"=w165:string)  [unwired: 13 in]
        n37 = Empty String/Path?(string/path=w177) -> (empty?=w175:bool)
        n38 = Not(x=w175) -> (.not. x?=w168:bool)
        n39 = And(x=w176, y=w168) -> (x .and. y?=w174:bool)
        n40 = Select(t="CheckRows", s=w174, f="Update: FilePath") -> (s? t:f=w169:string)
        n41 = call <vilib>:"Add State(s) to Queue__jki_lib_state_machine.vi"("State(s) in Front (\"\")"=w169, "State(s) in (\"\")"=w170) -> ("States Out"=w171:string)  [unwired: 13 in]
      }
      frame "CheckRows" {
        # "获取表格行里面，最新的测试结果保存到那一列了，新增加的测试结果就依次往后面添加。"
        # "仅select测试结果列"
        n42 = Array Size(array=w194) -> (size(s)=w203:i32)
        n43 = Search 1D Array(1D array=w194, element="T1") -> (index of element=w196:i32)  [unwired: 1 in]
        n44 = Index Array(array=w194, index #1=1 ("index")) -> (element #1=w225:string, element #2=w226:string, element #3=w206:string)  [unwired: 2 in]
        n45 = Build Array(w225, w226, w206) -> (w223:string[])
        n46 = Build Array("0" ("element"), w219, w218) -> (w222:string[])
        n47 = Subtract(x=w203, y=w196) -> (x-y=w202:i32)
        n48 = Array Subset(array=w194, index=w196, length=w202) -> (w201:string[])
        n49 = call <userlib>:"SQL_Select From DB Table.vi"("DB Type"=T2."SQLite", "SelectedColumnsNameList"=w201, "ColumnsValue"=w222, "ColumnsNameList"=w223, "TableName"=w220) -> ("Select SQL CMD"=w208:string)  [unwired: 6 in]
        n50 = call-dynamic "SQL Execute.vi"("error in (no error)"=w213, "Command Text"=w208, "HostDB in"=w217) -> ("error out"=w212:errorcluster, "FirstRow"=w199:string[], "HostDB out"=w216:refnum<class "SQLite.lvclass">)  [unwired: 4 in, 2 out]
        "FirstRow" <- w199
        n51 = for {
          tunnel: w199 -> [w231] mode=indexing
          tunnel: [w227] -> w195
          i -> [w227]
          stop <- w228 stop-if-true
          n52 = String Length(string=w231) -> (length=w230:i32)
          n53 = Less?(x=w230, y=1) -> (x < y?=w228:bool)
        }
        "EmptyResultColumnIndex" <- w195
        n54 = call <vilib>:"Add State(s) to Queue__jki_lib_state_machine.vi"("State(s) in Front (\"\")"=w207, "State(s) in (\"\")"=w208) -> ("States Out"=w209:string)  [unwired: 13 in]
        n55 = call <vilib>:"Add State(s) to Queue__jki_lib_state_machine.vi"("State(s) in (\"\")"=w210, "State(s) at Back (\"\")"=w209) -> ("States Out"=w211:string)  [unwired: 13 in]
        n56 = Bundle By Name(cluster=w200, "ResultStartindex"=w196, "EmptyResultColumnIndex"=w195) -> (w197:T1)
        n57 = call <vilib>:"Add State(s) to Queue__jki_lib_state_machine.vi"("State(s) in Front (\"\")"="Update" ("State(s) in Front (\"\")"), "State(s) in (\"\")"=w214) -> ("States Out"=w215:string)  [unwired: 13 in]
      }
      frame "CheckDBRef" {
        n58 = property class="SQLite.lvclass"(reference=w255) -> (reference out=w234:refnum<class "SQLite.lvclass">, "Property:Table_ColunmsList"=w232:string[])  [unwired: 1 in, 1 out]
        n59 = Array Size(array=w232) -> (size(s)=w244:i32)
        n60 = Search 1D Array(1D array=w232, element="T1") -> (index of element=w242:i32)  [unwired: 1 in]
        n61 = Index Array(array=w232, index #1=1 ("index")) -> (element #1=w263:string, element #2=w264:string, element #3=w247:string)  [unwired: 2 in]
        n62 = Build Array(w263, w264, w247) -> (w261:string[])
        n63 = Build Array("0" ("element"), w257, w256) -> (w260:string[])
        n64 = Subtract(x=w244, y=w242) -> (x-y=w243:i32)
        n65 = Array Subset(array=w232, index=w242, length=w243) -> (w236:string[])
        n66 = call <userlib>:"SQL_Select From DB Table.vi"("DB Type"=T2."SQLite", "SelectedColumnsNameList"=w236, "ColumnsValue"=w260, "ColumnsNameList"=w261, "TableName"=w258) -> ("Select SQL CMD"=w248:string)  [unwired: 6 in]
        n67 = call-dynamic "SQL Execute.vi"("error in (no error)"=w251, "Command Text"=w248, "HostDB in"=w234) -> ("error out"=w240:errorcluster, "HostDB out"=w254:refnum<class "SQLite.lvclass">)  [unwired: 4 in, 3 out]
        n68 = case shown="No Error" w240 {
          selector: w240 -> [_ w272]
          tunnel: w239 -> [_ w273]
          tunnel: ["CheckResultNameList" ("TableName") w271] -> w237
          tunnel: w238 -> [_ w268]
          frame No Error {
            (unwired) "CheckRows" ("TableName")
          }
          frame Error {
            n69 = Unbundle By Name(w272) -> ("status"=w270:bool)
            n70 = Equal?(x=w268, y=0) -> (x = y?=w266:bool)
            n71 = And(x=w270, y=w266) -> (x .and. y?=w269:bool)
            n72 = call <vilib>:"Add State(s) to Queue__jki_lib_state_machine.vi"("State(s) in Front (\"\")"="Initialize" ("Remaining States"), "State(s) in (\"\")"=w273) -> ("States Out"=w274:string)  [unwired: 13 in]
            n73 = Select(t=w274, s=w269, f="") -> (s? t:f=w271:string)
          }
        }
        n74 = call <vilib>:"Clear Errors.vi"("error in (no error)"=w240) -> ("error out"=w235:errorcluster)  [unwired: 5 in, 1 out]
        n75 = call <vilib>:"Add State(s) to Queue__jki_lib_state_machine.vi"("State(s) in (\"\")"=w249) -> ("States Out"=w250:string)  [unwired: 14 in]
        n76 = call <vilib>:"Add State(s) to Queue__jki_lib_state_machine.vi"("State(s) in Front (\"\")"=w237, "State(s) in (\"\")"=w252) -> ("States Out"=w253:string)  [unwired: 13 in]
      }
      frame "CheckResultNameList" {
        # "更新新的列名称alais到ColumnName这一行。"
        n77 = property class="SQLite.lvclass"(reference=w309) -> (reference out=w302:refnum<class "SQLite.lvclass">, "Property:Alais_ColunmsList"=w290:string[], "Property:Table_ColunmsList"=w289:string[])  [unwired: 1 in, 1 out]
        n78 = call <userlib>:"StringToArray_Sushu.vi"("State Queue"=w285) -> ("Array"=w305:string[])  [unwired: 7 in, 3 out]
        n79 = Search 1D Array(1D array=w289, element="Result") -> (index of element=w303:i32)  [unwired: 1 in]
        n80 = Array Size(array=w290) -> (size(s)=w288:i32)
        n81 = for {
          tunnel: w305 -> [w326] mode=indexing
          tunnel: w290 -> [w330]
          tunnel: w303 -> [w329]
          tunnel: [w326] -> w281 mode=indexing if=w325
          n82 = Search 1D Array(1D array=w330, element=w326, start index (0)=w329) -> (index of element=w328:i32)
          n83 = Equal?(x=w328, y=-1) -> (x = y?=w325:bool)
        }
        n84 = Index Array(array=w289, index #1=1 ("index")) -> (element #1=w299:string, element #2=w298:string)  [unwired: 1 in]
        n85 = Array Size(array=w281) -> (size(s)=w287:i32)
        n86 = Build Array(w299, w298) -> (w297:string[])
        n87 = Build Array("0" ("element"), "ColumnName" ("element")) -> (w295:string[])
        n88 = Array Subset(array=w289, index=w288, length=w287) -> (w286:string[])
        n89 = Empty Array?(array=w281) -> (empty?=w280:bool)
        n90 = call <userlib>:"Build string_ColumnsName=ColumnsValue_Where and.vi"("DB Type"=T2."SQLite", "ColumnsValue"=w295, "Check ASCII?"=FALSE, "ColumnsNameList"=w297) -> ("ColumnName='ColumnValue'"=w292:string)  [unwired: 7 in]
        n91 = case shown="True" w280 {
          tunnel: w302 -> [w320 w324]
          tunnel: w301 -> [w319 w323]
          tunnel: w292 -> [w318 _]
          tunnel: w286 -> [w317 _]
          tunnel: [w315 w324] -> w284
          tunnel: [w313 w323] -> w283
          tunnel: w282 -> [w312 _]
          tunnel: w281 -> [w311 _]
          frame False {
            n92 = call <userlib>:"SQL_Update DB Table.vi"("where name='value'"=w318, "ColumnsValue"=w311, "ColumnsNameList"=w317, "TableName"=w312) -> ("Update CMD"=w321:string)  [unwired: 7 in]
            "Update CMD 2" <- w321
            n93 = call-dynamic "SQL Execute.vi"("error in (no error)"=w319, "Return Data (T)"=FALSE, "Command Text"=w321, "HostDB in"=w320) -> ("error out"=w314:errorcluster, "HostDB out"=w316:refnum<class "SQLite.lvclass">)  [unwired: 3 in, 3 out]
            n94 = call-dynamic "Get Table Columns Name.vi"("error in (no error)"=w314, "TableName"=w312, "HostDB in"=w316) -> ("error out"=w313:errorcluster, "HostDB out"=w315:refnum<class "SQLite.lvclass">)  [unwired: 4 in, 3 out]
          }
          frame True {
          }
        }
        n95 = call <vilib>:"Add State(s) to Queue__JKI_lib_State_Machine.vi"("State(s) in Front (\"\")"="UpdateNewResult" ("State(s) in Front (\"\")"), "State(s) in (\"\")"=w278) -> ("States Out"=w279:string)  [unwired: 13 in]
      }
      frame "UpdateNewResult" {
        # "更新新的列名称alais到ColumnName这一行。"
        n96 = property class="SQLite.lvclass"(reference=w370) -> (reference out=w363:refnum<class "SQLite.lvclass">, "Property:Alais_ColunmsList"=w361:string[], "Property:Table_ColunmsList"=w333:string[])  [unwired: 1 in, 1 out]
        n97 = call <userlib>:"StringToArray_Sushu.vi"("State Queue"=w360) -> ("Array"=w366:string[])  [unwired: 7 in, 3 out]
        n98 = call <userlib>:"StringToArray_Sushu.vi"("State Queue"=w350) -> ("Array"=w349:string[])  [unwired: 7 in, 3 out]
        n99 = Search 1D Array(1D array=w333, element="Result") -> (index of element=w364:i32)  [unwired: 1 in]
        n100 = Build Array (concatenate)(w348, w349) -> (w347:string[])
        n101 = for {
          tunnel: w366 -> [w375] mode=indexing
          tunnel: w361 -> [w377]
          tunnel: w364 -> [w376]
          tunnel: w333 -> [w374]
          tunnel: [w372] -> w345 mode=indexing
          n102 = Search 1D Array(1D array=w377, element=w375, start index (0)=w376) -> (index of element=w373:i32)
          n103 = Index Array(array=w374, index=w373) -> (element=w372:string)
        }
        n104 = Index Array(array=w333, index #1=1 ("index")) -> (element #1=w342:string, element #2=w341:string, element #3=w340:string)  [unwired: 2 in]
        n105 = Build Array("0" ("element"), w332, w331) -> (w337:string[])
        n106 = Build Array(w342, w341, w340) -> (w339:string[])
        n107 = call <userlib>:"Build string_ColumnsName=ColumnsValue_Where and.vi"("DB Type"=T2."SQLite", "ColumnsValue"=w337, "Check ASCII?"=FALSE, "ColumnsNameList"=w339) -> ("ColumnName='ColumnValue'"=w334:string)  [unwired: 7 in]
        n108 = Build Array (concatenate)("Result" ("TableName"), w345) -> (w346:string[])
        n109 = call <userlib>:"SQL_Update DB Table.vi"("where name='value'"=w334, "ColumnsValue"=w347, "ColumnsNameList"=w346, "TableName"=w357) -> ("Update CMD"=w353:string)  [unwired: 7 in]
        "Update CMD 3" <- w353
        n110 = call-dynamic "SQL Execute.vi"("error in (no error)"=w362, "Return Data (T)"=FALSE, "Command Text"=w353, "HostDB in"=w363) -> ("error out"=w351:errorcluster, "HostDB out"=w352:refnum<class "SQLite.lvclass">)  [unwired: 3 in, 3 out]
        n111 = call-dynamic "Get Table Columns Name.vi"("error in (no error)"=w351, "TableName"=w357, "HostDB in"=w352) -> ("error out"=w358:errorcluster, "HostDB out"=w359:refnum<class "SQLite.lvclass">)  [unwired: 4 in, 3 out]
        n112 = call <vilib>:"Add State(s) to Queue__jki_lib_state_machine.vi"("State(s) in (\"\")"=w355) -> ("States Out"=w356:string)  [unwired: 14 in]
      }
      frame "Update" {
        n113 = Unbundle By Name(w392) -> ("ResultStartindex"=w391:i32, "EmptyResultColumnIndex"=w390:i32)
        n114 = Index Array(array=w383, index #1=1 ("index")) -> (element #1=w406:string, element #2=w405:string, element #3=w404:string)  [unwired: 2 in]
        n115 = call <userlib>:"StringToArray_Sushu.vi"("State Queue"=w393) -> ("Array"=w387:string[], "Final size(s)"=w386:i32)  [unwired: 7 in, 2 out]
        n116 = Build Array("0" ("element"), w415, w414) -> (w401:string[])
        n117 = Build Array(w406, w405, w404) -> (w403:string[])
        n118 = Add(x=w391, y=w390) -> (x+y=w388:i32)
        n119 = Array Subset(array=w383, index=w388, length=w386) -> (w389:string[])
        n120 = call <userlib>:"Build string_ColumnsName=ColumnsValue_Where and.vi"("DB Type"=T2."SQLite", "ColumnsValue"=w401, "Check ASCII?"=FALSE, "ColumnsNameList"=w403) -> ("ColumnName='ColumnValue'"=w408:string)  [unwired: 7 in]
        n121 = Build Array (concatenate)(w380, w387) -> (w381:string[])
        n122 = Build Array (concatenate)("Result" ("Name"), w389) -> (w379:string[])
        n123 = call <userlib>:"SQL_Update DB Table.vi"("where name='value'"=w408, "ColumnsValue"=w381, "ColumnsNameList"=w379, "TableName"=w416) -> ("Update CMD"=w395:string)  [unwired: 7 in]
        "Update CMD" <- w395
        n124 = call-dynamic "SQL Execute.vi"("error in (no error)"=w385, "Return Data (T)"=FALSE, "Command Text"=w395, "HostDB in"=w413) -> ("error out"=w384:errorcluster, "HostDB out"=w412:refnum<class "SQLite.lvclass">)  [unwired: 3 in, 3 out]
        n125 = call <vilib>:"Add State(s) to Queue__jki_lib_state_machine.vi"("State(s) in (\"\")"=w409) -> ("States Out"=w410:string)  [unwired: 14 in]
        n126 = call <vilib>:"Add State(s) to Queue__jki_lib_state_machine.vi"("State(s) in Front (\"\")"=w394, "State(s) in (\"\")"=w395) -> ("States Out"=w396:string)  [unwired: 13 in]
        n127 = call <vilib>:"Add State(s) to Queue__jki_lib_state_machine.vi"("State(s) in (\"\")"=w397, "State(s) at Back (\"\")"=w396) -> ("States Out"=w398:string)  [unwired: 13 in]
      }
      frame "Close" {
        n128 = call-dynamic "Close Connection.vi"("error in (no error)"=w420, "HostDB in"=w418) -> ("error out"=w419:errorcluster, "HostDB out"=w417:refnum<class "SQLite.lvclass">)  [unwired: 8 in]
      }
    }
  }
  "error out" <- w3
  "CMD" <- w7
  n129 = Random Number (0-1)() -> (number: 0 to 1=→"number (0 to 1)":dbl)
